vi "Create Base.vi"(9 "jettl":refnum<class "jettl.lvclass">, 10 "Self Alias":string) -> (2 "jettl":refnum<class "jettl.lvclass">)   [LabVIEW 2021, in "jettl.lvlib"]
uses:
  jettl.lvlib
  Addresses Strategy/Addresses Strategy.lvlib
  Base jettl/Base jettl.lvclass
  Msg Strategy/Msg Strategy.lvclass
  C:/git/jettl/jettl/jettl/jettl/jettl.lvclass
  C:/git/jettl/jettl/Create Msg Strategy/Create/Create.lvclass
  C:/git/jettl/jettl/jettl/Last Ack Msg Strategy/Last Ack/Last Ack.lvclass
  C:/git/jettl/jettl/Merge Error Msg Strategy/Merge Error/Merge Error.lvclass
  C:/git/jettl/jettl/Override Error Msg Strategy/Override Error/Override Error.lvclass
  C:/git/jettl/jettl/Setup Msg Strategy/Setup/Setup.lvclass
  C:/git/jettl/jettl/Teardown Msg Strategy/Teardown/Teardown.lvclass
  C:/git/jettl/jettl/jettl/Base jettl/Base jettl.lvclass
  jettl/jettl.lvclass
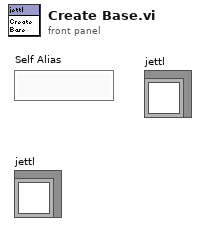
[diagram p1: front panel]
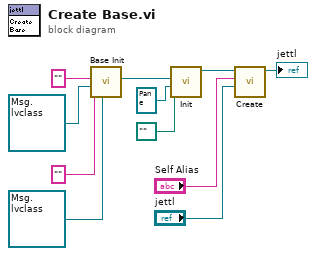
[diagram p0: block diagram]
diagram:
  n1 = call "Base Init.vi"("Creator"=refnum<user-event> refnum, "Creator Alias"="", "Self"=refnum<user-event> refnum, "Self Alias"="") -> ("Addresses Strategy out"=w7:refnum<class "Addresses Strategy.lvclass">)  [unwired: 7 in]
  n2 = call "Init.vi"("Path"=path "", "Register"=refnum<event-registration> refnum, "Addresses Strategy"=w7) -> ("Base jettl out"=w8:refnum<class "Base jettl.lvclass">)  [unwired: 8 in]
  n3 = call-dynamic "Create.vi"("jettl"="jettl", "Self Alias"="Self Alias", "Base jettl in"=w8) -> ("Base jettl out"=→"jettl":refnum<class "Base jettl.lvclass">)  [unwired: 8 in]
